vi "write_params.vi"(8 "error in (no error)":errorcluster, 10 "params":T1={"fit_intercept"=TRUE, "verbose"={"verbose_type"="bool", "verbose_bool"=FALSE, "verbose_int"=0.0}, "max_iter"=500.0, "normalize"=TRUE, "precompute"={"precompute_type"="auto", "precompute_bool"=FALSE, "precompute_list"=[]}, "cv"=5.0, "max_n_alphas"=1000.0, "n_jobs"=1.0, "copy_X"=TRUE, "positive"=FALSE}, 11 "LassoLarsCV in":refnum<class "LassoLarsCV.lvclass">) -> (0 "error out":errorcluster, 3 "LassoLarsCV out":refnum<class "LassoLarsCV.lvclass">)   [LabVIEW 2020, in "LassoLarsCV.lvclass"]
uses:
  LassoLarsCV.lvclass
  Controls/lasso_lars_cv_params.ctl
  LassoLarsCV.lvclass/LassoLarsCV.ctl
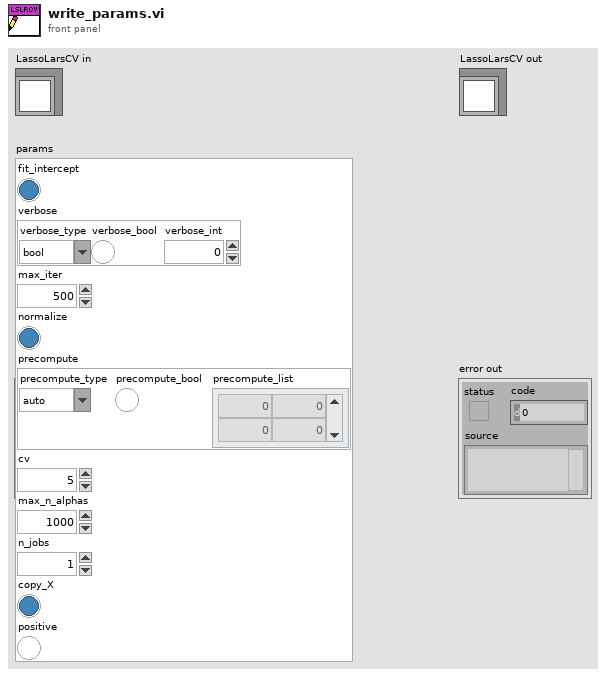
[diagram p1: front panel]
types:
  T1 = typedef "lasso_lars_cv_params.ctl" = cluster{"fit_intercept":bool, "verbose":cluster{"verbose_type":string, "verbose_bool":bool, "verbose_int":dbl}, "max_iter":dbl, "normalize":bool, "precompute":cluster{"precompute_type":string, "precompute_bool":bool, "precompute_list":dbl[][]}, "cv":dbl, "max_n_alphas":dbl, "n_jobs":dbl, "copy_X":bool, "positive":bool}
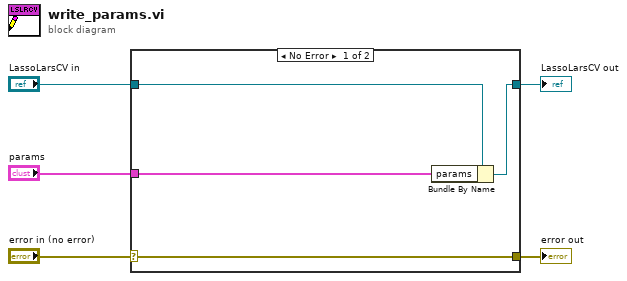
[diagram p0: block diagram]
diagram:
  n1 = case shown="No Error" "error in (no error)" {
    selector: "error in (no error)" -> [w9 w10]
    tunnel: [w9 w10] -> w4
    tunnel: [w7 w11] -> w2
    tunnel: "LassoLarsCV in" -> [w8 w11]
    tunnel: "params" -> [w6 _]
    frame No Error {
      n2 = Bundle By Name(cluster=w8, "params"=w6) -> (w7:refnum<class "LassoLarsCV.lvclass">)
    }
    frame Error {
    }
  }
  "error out" <- w4
  "LassoLarsCV out" <- w2
